vi "Parse Signal List.vi"(8 "error in":errorcluster, 11 "AnalogInput in":refnum<class "AnalogInput.lvclass">) -> (0 "error out":errorcluster, 3 "AnalogInput out":refnum<class "AnalogInput.lvclass">)   [LabVIEW 2019, in "AnalogInput.lvlib" / "AnalogInput.lvclass"]
uses:
  Library/AnalogInput.lvclass
  C:/Users/Public/Documents/Development/builds/Tools/Config.lvlibp/Config.lvclass
  Custom Controls/Signal Keys.ctl
  Library/AnalogInput.lvclass/AnalogInput.ctl
  builds/Tools/Config.lvlibp/Accessors/Read Device Signals.vi
panel:
  in  "Signal Keys":T1
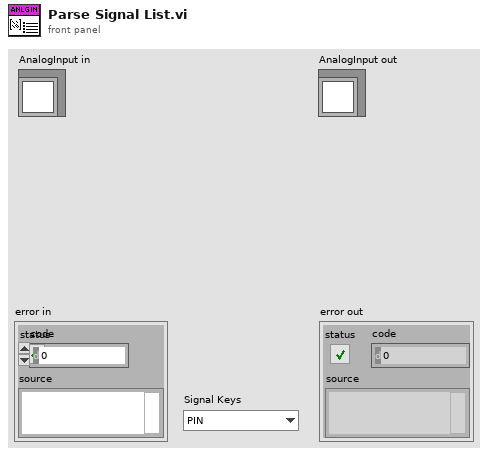
[diagram p1: front panel]
types:
  T1 = typedef "AnalogInput.lvlib/AnalogInput.lvclass/Signal Keys.ctl" = enum16{"PIN", "NAME", "MIN", "MAX", "TRIG_NAME", "TRIG_SRC"}
  T2 = typedef "AnalogInput.lvlib/AnalogInput.lvclass/Range.ctl" = cluster{"Max Value":dbl, "Min Value":dbl}
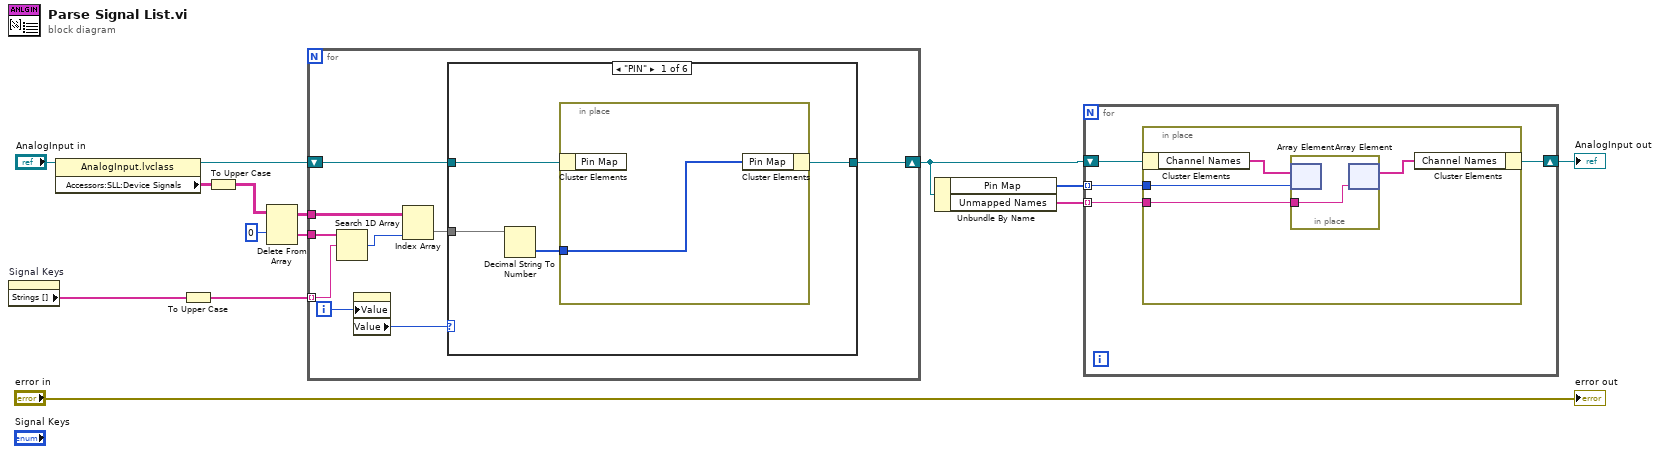
[diagram p0: block diagram]
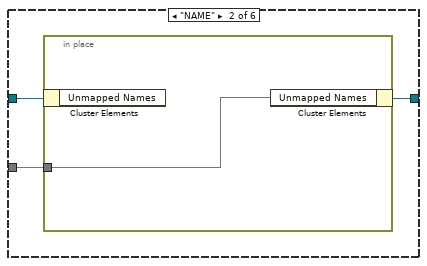
[diagram p2: hidden frame]
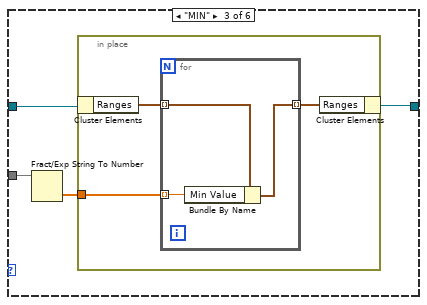
[diagram p3: hidden frame]
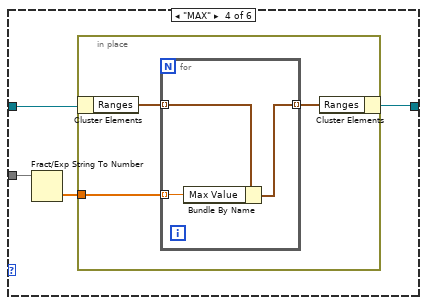
[diagram p4: hidden frame]
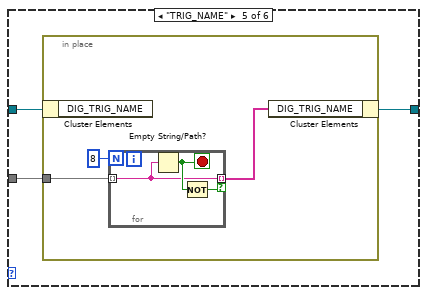
[diagram p5: hidden frame]
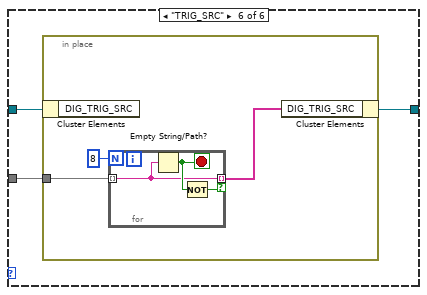
[diagram p6: hidden frame]
diagram:
  n1 = property on="Signal Keys" class="Enum (strict)"() -> ("Strings []"=w12:string[])  [unwired: 2 in, 2 out]
  n2 = property class="AnalogInput.lvclass"(reference="AnalogInput in") -> (reference out=w9:refnum<class "AnalogInput.lvclass">, "Accessors:SLL:Device Signals"=w8:string[][])  [unwired: 1 in, 1 out]
  n3 = To Upper Case(1:w12) -> (0:w1:string[])
  n4 = To Upper Case(1:w8) -> (0:w2:string[][])
  n5 = Delete From Array(array=w2, index (row)=0) -> (deleted portion=w3:string[], array with subset deleted=w10:string[][])  [unwired: 2 in]
  n6 = for {
    tunnel: w1 -> [w16] mode=indexing
    shift-right: [w18] -> w7
    shift-left: w9 -> [w19]
    tunnel: w10 -> [w22]
    tunnel: w3 -> [w17]
    i -> [w23]
    n7 = Search 1D Array(1D array=w17, element=w16) -> (index of element=w15:i32)  [unwired: 1 in]
    n8 = property on="Signal Keys" class="Enum (strict)"("Value"=w23) -> ("Value"=w21:T1)  [unwired: 2 in, 2 out]
    n9 = Index Array(array=w22, index (col)=w15) -> (element=w20:string[])  [unwired: 1 in]
    n10 = case shown="\"PIN\"" w21 {
      tunnel: w20 -> [w27 w29 w34 w44 w53 w62]
      tunnel: w19 -> [w26 w31 w36 w46 w55 w64]
      tunnel: [w24 w30 w35 w45 w54 w63] -> w18
      frame "PIN" {
        n11 = Decimal String To Number(string=w27) -> (number=w25:i32[])  [unwired: 2 in, 1 out]
        n12 = in-place {
          in-place-border: w25 -> [w28]
          n13 = in-place-cluster #1(w26) -> ()  [unwired: 1 out]
          n14 = in-place-cluster #1("Pin Map"=w28) -> (w24:refnum<class "AnalogInput.lvclass">)
        }
      }
      frame "NAME" {
        n15 = in-place {
          in-place-border: w29 -> [w32]
          n16 = in-place-cluster #2(w31) -> ()  [unwired: 1 out]
          n17 = in-place-cluster #2("Unmapped Names"=w32) -> (w30:refnum<class "AnalogInput.lvclass">)
        }
      }
      frame "MIN" {
        n18 = Fract/Exp String To Number(string=w34) -> (number=w33:dbl[])  [unwired: 3 in, 1 out]
        n19 = in-place {
          in-place-border: w33 -> [w37]
          n20 = in-place-cluster #3(w36) -> ("Ranges"=w39:T2[])
          n21 = for {
            tunnel: w39 -> [w42] mode=indexing
            tunnel: [w41] -> w38 mode=indexing
            tunnel: w37 -> [w40] mode=indexing
            n22 = Bundle By Name(cluster=w42, "Min Value"=w40) -> (w41:T2)
          }
          n23 = in-place-cluster #3("Ranges"=w38) -> (w35:refnum<class "AnalogInput.lvclass">)
        }
      }
      frame "MAX" {
        n24 = Fract/Exp String To Number(string=w44) -> (number=w43:dbl[])  [unwired: 3 in, 1 out]
        n25 = in-place {
          in-place-border: w43 -> [w47]
          n26 = in-place-cluster #4(w46) -> ("Ranges"=w49:T2[])
          n27 = for {
            tunnel: w49 -> [w52] mode=indexing
            tunnel: [w51] -> w48 mode=indexing
            tunnel: w47 -> [w50] mode=indexing
            n28 = Bundle By Name(cluster=w52, "Max Value"=w50) -> (w51:T2)
          }
          n29 = in-place-cluster #4("Ranges"=w48) -> (w45:refnum<class "AnalogInput.lvclass">)
        }
      }
      frame "TRIG_NAME" {
        n30 = in-place {
          in-place-border: w53 -> [w57]
          n31 = in-place-cluster #5(w55) -> ()  [unwired: 1 out]
          n32 = for {
            N: 8 -> [_]
            tunnel: w57 -> [w59] mode=indexing
            tunnel: [w59] -> w56 mode=indexing if=w60
            stop <- w61 stop-if-true
            n33 = Empty String/Path?(string/path=w59) -> (empty?=w61:bool)
            n34 = Not(x=w61) -> (.not. x?=w60:bool)
          }
          n35 = in-place-cluster #5("DIG_TRIG_NAME"=w56) -> (w54:refnum<class "AnalogInput.lvclass">)
        }
      }
      frame "TRIG_SRC" {
        n36 = in-place {
          in-place-border: w62 -> [w66]
          n37 = in-place-cluster #6(w64) -> ()  [unwired: 1 out]
          n38 = for {
            N: 8 -> [_]
            tunnel: w66 -> [w68] mode=indexing
            tunnel: [w68] -> w65 mode=indexing if=w69
            stop <- w70 stop-if-true
            n39 = Empty String/Path?(string/path=w68) -> (empty?=w70:bool)
            n40 = Not(x=w70) -> (.not. x?=w69:bool)
          }
          n41 = in-place-cluster #6("DIG_TRIG_SRC"=w65) -> (w63:refnum<class "AnalogInput.lvclass">)
        }
      }
    }
  }
  n42 = Unbundle By Name(w7) -> ("Pin Map"=w5:i32[], "Unmapped Names"=w4:string[])
  n43 = for {
    shift-right: [w72] -> w6
    shift-left: w7 -> [w73]
    tunnel: w4 -> [w71] mode=indexing
    tunnel: w5 -> [w74] mode=indexing
    n44 = in-place {
      in-place-border: w74 -> [w78]
      in-place-border: w71 -> [w77]
      n45 = in-place-cluster #7(w73) -> ("Channel Names"=w76:string[])
      n46 = in-place {
        in-place-border: w77 -> [w79]
        n47 = in-place-array #8(w76, w78) -> ()  [unwired: 1 out]
        n48 = in-place-array #8(w79) -> (w75:string[])  [unwired: 1 out]
      }
      n49 = in-place-cluster #7("Channel Names"=w75) -> (w72:refnum<class "AnalogInput.lvclass">)
    }
  }
  "AnalogInput out" <- w6
  "error out" <- "error in"
